vi "Open and Run VI.vi"(6 "State (Hidden)":T1(ring)=enum."Hidden", 8 "error in (no error)":errorcluster, 10 "Run? (T)":bool=TRUE, 11 "vi path":path=path "C:/ARIES/LV/Libraries/AOS/SubVI/M2ES.vi") -> (0 "error out":errorcluster, 2 "Front Panel Window Was Open?":bool, 3 "VI":refnum<vi>)   [LabVIEW 2015, in "Utility.lvlib"]
doc: "This VI is used to dynamically open and run (if desired) another VI.\n\nThe initial state of the window can be specified (defaults to hidden).\n\nNote: in the development environment the absolute input path is used, however in the run-time system only the tail section of the filename is used. The file must be included in the build as a dynamic VI otherwise a run-time error will be generated."
uses:
  Utility.lvlib
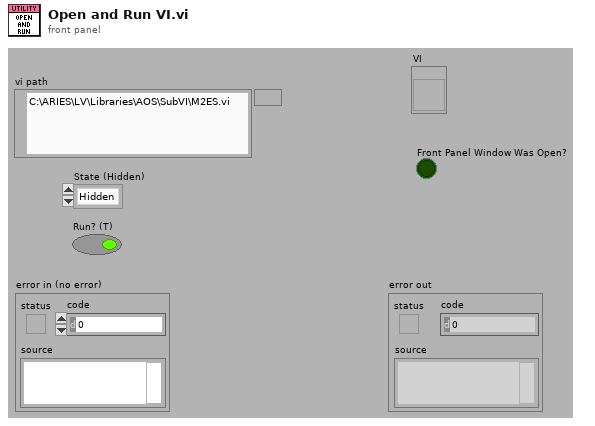
[diagram p1: front panel]
types:
  T1 = enum32{"Invalid", "Standard", "Closed", "Hidden", "Minimized", "Maximized"}
  T2 = enum32{"invalid app kind", "Development System", "Run Time System", "Student Edition", "Embedded LabVIEW", "Evaluation", "Custom"}
  T3 = enum32{"Bad", "Idle", "Run top level", "Running"}
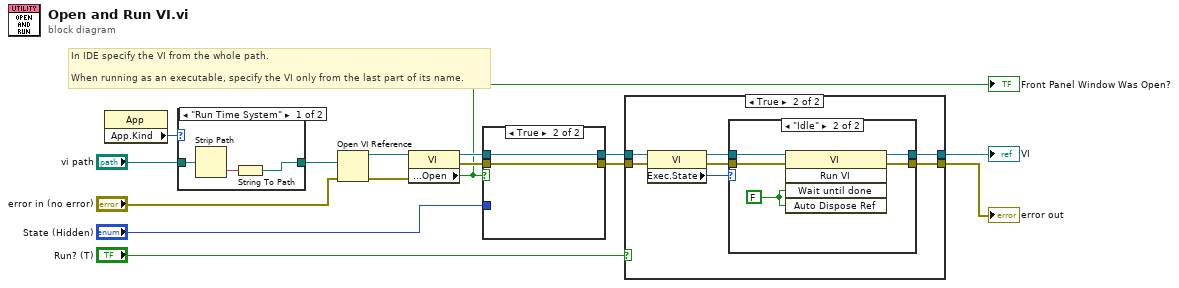
[diagram p0: block diagram]
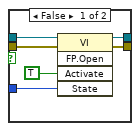
[diagram p2: hidden frame]
diagram:
  # "In IDE specify the VI from the whole path.\n\nWhen running as an executable, specify the VI only from the last part of its name."
  n1 = property class="App"() -> ("App.Kind"=w8:T2)  [unwired: 2 in, 2 out]
  n2 = case shown="\"Run Time System\"" w8 {
    tunnel: "vi path" -> [w18 w19]
    tunnel: [w16 w19] -> w1
    frame "Run Time System" {
      n3 = Strip Path(path=w18) -> (name=w17:string)  [unwired: 1 out]
      n4 = String To Path(string=w17) -> (path=w16:path)
    }
    frame Default {
    }
  }
  n5 = Open VI Reference(vi path=w1, error in (no error)="error in (no error)") -> (vi reference=w2:refnum<vi>, error out=w5:errorcluster)  [unwired: 1 in, 3 out]
  n6 = property class="VI"(reference=w2, error in=w5) -> (reference out=w6:refnum<vi>, error out=w4:errorcluster, "Front Panel.Open"=w3:bool)
  "Front Panel Window Was Open?" <- w3
  n7 = case shown="True" w3 {
    tunnel: "State (Hidden)" -> [w24 _]
    tunnel: [w23 w27] -> w13
    tunnel: [w22 w26] -> w12
    tunnel: w6 -> [w21 w27]
    tunnel: w4 -> [w20 w26]
    frame False {
      n8 = invoke class="VI" method="FP.Open"(reference=w21, error in=w20, "Activate"=TRUE ("Activate?"), "State"=w24) -> (reference out=w23:refnum<vi>, error out=w22:errorcluster)  [unwired: 1 in, 3 out]
    }
    frame True {
    }
  }
  n9 = case shown="True" "Run? (T)" {
    tunnel: w13 -> [w29 w34]
    tunnel: w12 -> [w28 w32]
    tunnel: [w28 w36] -> w11
    tunnel: [w29 w35] -> w10
    frame False {
    }
    frame True {
      n10 = property class="VI"(reference=w34, error in=w32) -> (reference out=w33:refnum<vi>, error out=w31:errorcluster, "Exec.State"=w30:T3)
      n11 = case shown="\"Idle\"" w30 {
        tunnel: [w37 w43] -> w36
        tunnel: [w38 w41] -> w35
        tunnel: w33 -> [w38 w40]
        tunnel: w31 -> [w37 w39]
        frame Default {
          # "Cannot run VI\n(perhaps it is already running)"
        }
        frame "Idle" {
          w42 = FALSE ("Wait Until Done")
          n12 = invoke class="VI" method="Run VI"(reference=w40, error in=w39, "Wait until done"=w42, "Auto Dispose Ref"=w42) -> (reference out=w41:refnum<vi>, error out=w43:errorcluster)  [unwired: 1 in, 3 out]
        }
      }
    }
  }
  "VI" <- w10
  "error out" <- w11
